vi "Test_RequestSynchronousData_RequestMultiple_OnePublished_TimeoutNonblocking.vi"(8 "error in (no error)":errorcluster, 11 "TestCase in":refnum<class "TestRequestSynchronousData.lvclass">) -> (0 "error out":errorcluster, 3 "TestCase out":refnum<class "TestRequestSynchronousData.lvclass">)   [LabVIEW 2020, in "TestRequestSynchronousData.lvclass"]
uses:
  TestRequestSynchronousData.lvclass
  TestRequestSynchronousData.lvclass/TestRequestSynchronousData.ctl
  24bf8875-c008-4f22-9bfa-88e42476d167.vi
  Source/IModel/IModel/IModel.lvclass
  Doubles/RootModelPublishesDoubleFloatX/RootModelPublishesDoubleFloatX.lvclass
  <vilib>/ActorFramework/Actor/Actor.lvclass
  Source/Mediator/Mediator/Mediator.lvclass
  <vilib>/ActorFramework/Stop Msg/Stop Msg.lvclass
  modules/composed-event-logger/Source/String Control Sink/String Control Sink.lvclass
  f7bee35d-b044-4098-91af-55574313c386.vi
  modules/composed-event-logger/Source/Composed Log/LoggerReference/LoggerReference.lvclass
  11850773-0e08-463b-84b0-7f64b956e994.vi
  Doubles/ModelSynchronouslyRequestsManyDoubleFloats/ModelSynchronouslyRequestsManyDoubleFloats.lvclass
  C:/Git/mva-core/Source/RootModel/RootModel/RootModel.lvclass
  C:/Git/mva-core/Source/IModel/IModel/IModel.lvclass
  C:/Git/mva-core/Source/IObserver/IObserver/IObserver.lvclass
  C:/Program Files (x86)/National Instruments/LabVIEW 2020/vi.lib/ActorFramework/Actor/Actor.lvclass
  C:/Git/mva-core/Test/Doubles/RootModelPublishesDoubleFloatX/RootModelPublishesDoubleFloatX.lvclass
  C:/Git/mva-core/Test/Doubles/ModelSynchronouslyRequestsManyDoubleFloats/ModelSynchronouslyRequestsManyDoubleFloats.lvclass
panel:
  out "Result":T1(array[cluster])
  out "Log":string
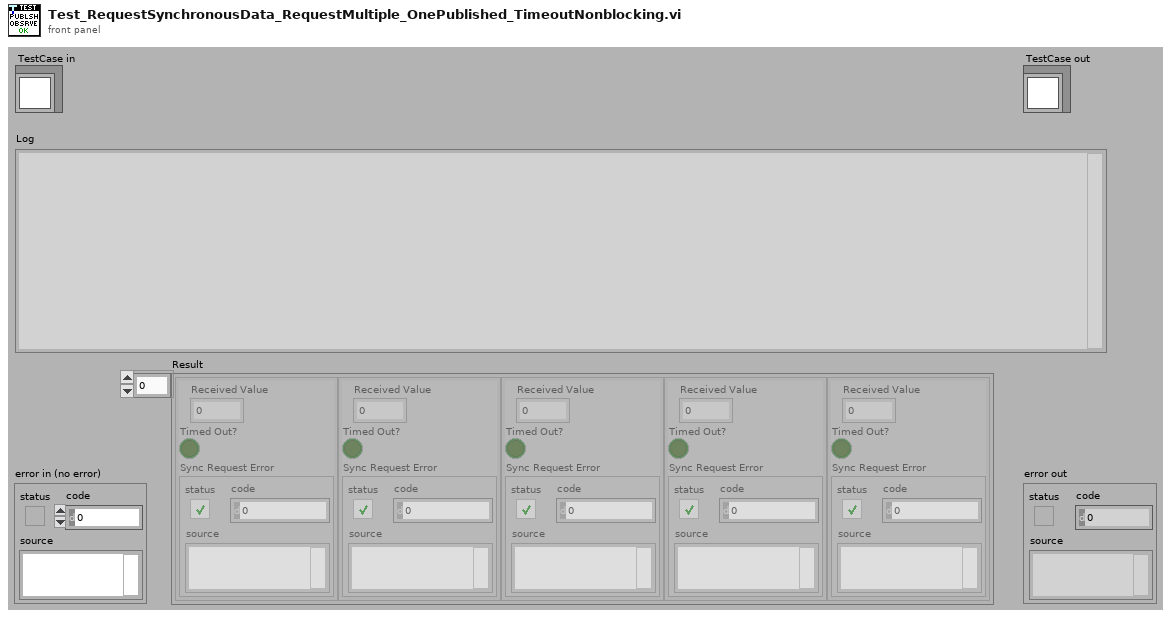
[diagram p1: front panel]
types:
  T1 = cluster{"Received Value":dbl, "Timed Out?":bool, "Sync Request Error":errorcluster}[]
  T2 = cluster{"Received Value":dbl, "Timed Out?":bool, "Sync Request Error":errorcluster}
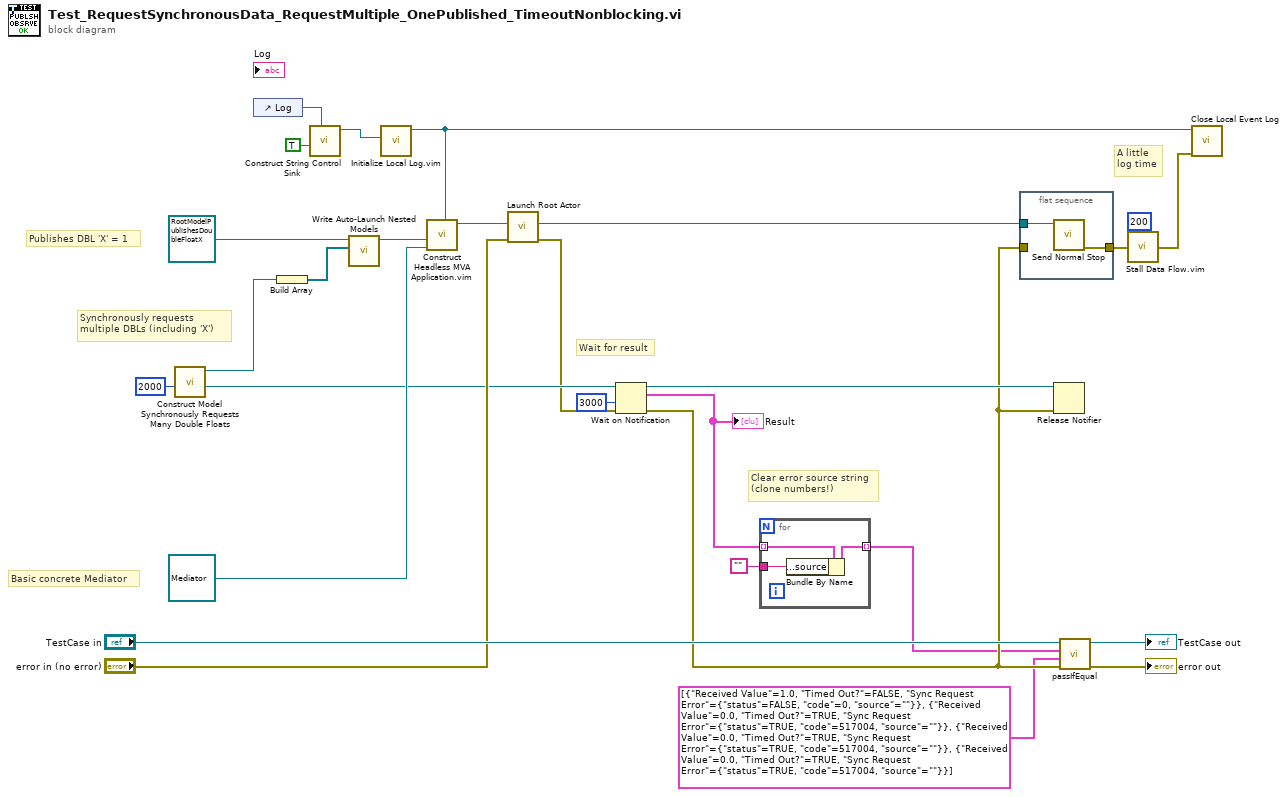
[diagram p0: block diagram]
diagram:
  # "Clear error source string\n(clone numbers!)"
  # "A little\nlog time"
  # "Wait for result"
  # "Basic concrete Mediator"
  # "Synchronously requests\nmultiple DBLs (including 'X')"
  # "Publishes DBL 'X' = 1"
  n1 = call "Construct Model Synchronously Requests Many Double Floats.vi"("DBL Request Timeout (2000)"=2000) -> ("Results Notifier"=w16:refnum<notifier>, "ModelSynchronouslyRequestsManyDoubleFloats Out"=w8:refnum<class "ModelSynchronouslyRequestsManyDoubleFloats.lvclass">)  [unwired: 9 in]
  n2 = control-ref of="Log"() -> (w15:refnum<vi>)
  n3 = Build Array(w8) -> (w24:refnum<class "ModelSynchronouslyRequestsManyDoubleFloats.lvclass">[])
  n4 = call "Construct String Control Sink.vi"("Str Refnum"=w15, "AutoScroll?(F)"=TRUE) -> ("String Control Sink out"=w14:refnum<class "String Control Sink.lvclass">)  [unwired: 9 in]
  n5 = call "Write Auto-Launch Nested Models.vi"("Auto-Launch Nested Models"=w24, "IModel In"=refnum<class "RootModelPublishesDoubleFloatX.lvclass"> refnum ("RootModelPublishesDoubleFloatX.lvclass")) -> ("IModel Out"=w23:refnum<class "RootModelPublishesDoubleFloatX.lvclass">)  [unwired: 9 in]
  n6 = call "Initialize Local Log.vim"("Startup Sink(s)"=w14) -> ("Log Instance Reference"=w12:refnum<class "LoggerReference.lvclass">)  [unwired: 8 in, 2 out]
  n7 = call "Construct Headless MVA Application.vim"("Parent Log Reference"=w12, "Mediator Type"=refnum<class "Mediator.lvclass"> refnum ("Mediator.lvlib:Mediator.lvclass"), "RootModel in"=w23) -> ("RootModel out"=w22:refnum<class "RootModelPublishesDoubleFloatX.lvclass">)  [unwired: 8 in]
  n8 = call <vilib>:"Launch Root Actor.vi"("error in (no error)"="error in (no error)", "Actor"=w22) -> ("error out"=w6:errorcluster, "Actor's Enqueuer"=w18:refnum<class "Message Enqueuer.lvclass">)  [unwired: 8 in]
  n9 = Wait on Notification(notifier=w16, timeout in ms (-1)=3000, error in (no error)=w6) -> (notifier out=w21:refnum<notifier>, notification=w3:T1, error out=w5:errorcluster)  [unwired: 1 in, 1 out]
  "Result" <- w3
  n10 = for {
    tunnel: w3 -> [w31] mode=indexing
    tunnel: [w30] -> w1 mode=indexing
    tunnel: "" -> [w29]
    n11 = Bundle By Name(cluster=w31, "Sync Request Error.source"=w29) -> (w30:T2)
  }
  n12 = flat-sequence {
    tunnel: w18 -> [w33]
    tunnel: [w32] -> w11
    tunnel: w5 -> [_]
    frame #0 {
      n13 = call <vilib>:"Send Normal Stop.vi"("Message Enqueuer"=w33) -> ("error out"=w32:errorcluster)  [unwired: 10 in]
    }
  }
  n14 = Release Notifier(notifier=w21, error in (no error)=w5) -> ()  [unwired: 1 in, 3 out]
  n15 = call-dynamic "passIfEqual.vi"("error in (no error)"=w5, "y"=T1 [{"Received Value"=1.0, "Timed Out?"=FALSE, "Sync Request Error"={"status"=FALSE, "code"=0, "source"=""}}, {"Received Value"=0.0, "Timed Out?"=TRUE, "Sync Request Error"={"status"=TRUE, "code"=517004, "source"=""}}, {"Received Value"=0.0, "Timed Out?"=TRUE, "Sync Request Error"={"status"=TRUE, "code"=517004, "source"=""}}, {"Received Value"=0.0, "Timed Out?"=TRUE, "Sync Request Error"={"status"=TRUE, "code"=517004, "source"=""}}] ("Result 2"), "x"=w1, "TestCase in"="TestCase in") -> ("error out"=→"error out":errorcluster, "TestCase out"=→"TestCase out":refnum<class "TestRequestSynchronousData.lvclass">)  [unwired: 6 in]
  n16 = call "Stall Data Flow.vim"("value in"=w11, "milliseconds to wait"=u32 200) -> ("value out"=w10:errorcluster)  [unwired: 1 out]
  n17 = call "Close Local Event Log.vi"("error in (no error)"=w10, "Log Instance"=w12) -> ()  [unwired: 9 in, 1 out]
